vi "TEST_Camera.vi"() -> ()   [LabVIEW 2018]
uses:
  <vilib>/vision/Image Controls.llb/IMAQ Image.ctl
  <vilib>/myRIO/Instrument Drivers/Onboard IO/UART/typedef/VISA Configuration.ctl
  <vilib>/myRIO/Common/Instrument Driver Framework/myRIO v1.0/UART/vis/myRIO v1.0 Close UART.vi
  <vilib>/Instr/_visa.llb/VISA Configure Serial Port (Instr).vi
  <vilib>/Utility/error.llb/Error Cluster From Error Code.vi
  <vilib>/myRIO/Common/Instrument Driver Framework/myRIO v1.0/DIO/vis/myRIO v1.0 Write DIO.vi
  <vilib>/myRIO/Common/Instrument Driver Framework/myRIO v1.0/PWM/vis/myRIO v1.0 Write PWM.vi
  <vilib>/myRIO/Common/Instrument Driver Framework/Utilities/vis/FPGA Ref Manager.vi
  <vilib>/myRIO/Common/Instrument Driver Framework/myRIO v1.0/myRIO v1.0 Reset FPGA.vi
  <vilib>/myRIO/Common/Instrument Driver Framework/myRIO v1.0/IRQ/vis/myRIO v1.0 IRQ Info FGV.vi
  <vilib>/myRIO/Common/Instrument Driver Framework/myRIO v1.0/IRQ/vis/myRIO v1.0 Timer IRQ Info FGV.vi
  <vilib>/myRIO/Common/Instrument Driver Framework/myRIO v1.0/IRQ/vis/myRIO v1.0 ISR Agent.vi
  <vilib>/myRIO/Instrument Drivers/Onboard IO/PWM/PWM.lvlib
  <vilib>/vision/driver/NI_Vision_Acquisition_Software.lvlib
  <vilib>/vision/NI_Vision_Development_Module.lvlib
  <vilib>/myRIO/Instrument Drivers/Utilities/Utilities.lvlib
  <vilib>/myRIO/Instrument Drivers/Onboard IO/DIO/DIO.lvlib
  <vilib>/myRIO/Instrument Drivers/Onboard IO/UART/UART.lvlib
panel:
  in  "RollDetect":bool
  in  "RtF":bool
  in  "State ind":bool
  out "Character Count":u32
  in  "Grounded?":bool
  out "Image 7":T1(plugin-control)
  out "Image Pixels (U8)":u8[][](array[numeric])
  out "Image 6":T1(plugin-control)
  in  "Stop":bool
  out "Image 5":T1(plugin-control)
  out "Y":dbl[](array[numeric])
  out "X":dbl[](array[numeric])
  out "Antal isbjerg":i32
  out "logfile name":path
  in  "logfile base name":string="logfile"
  in  "Color Plane (Color Plane Extraction 1)":i32(ring)=1 items=["Red", "Green", "Blue", "Hue", "Saturation", "Luminance", "Value", "Intensity"]
  in  "Range (Threshold 1)":cluster{"Lower value":sgl, "Upper value":sgl}={"Lower value"=230.0, "Upper value"=255.0}
  in  "Structuring Element (Basic Morphology 1)":i32[][](array[numeric])=[[0, 1, 0], [1, 1, 1], [0, 1, 0]]
  in  "Number of Erosion (Advanced Morphology 1)":i32=12
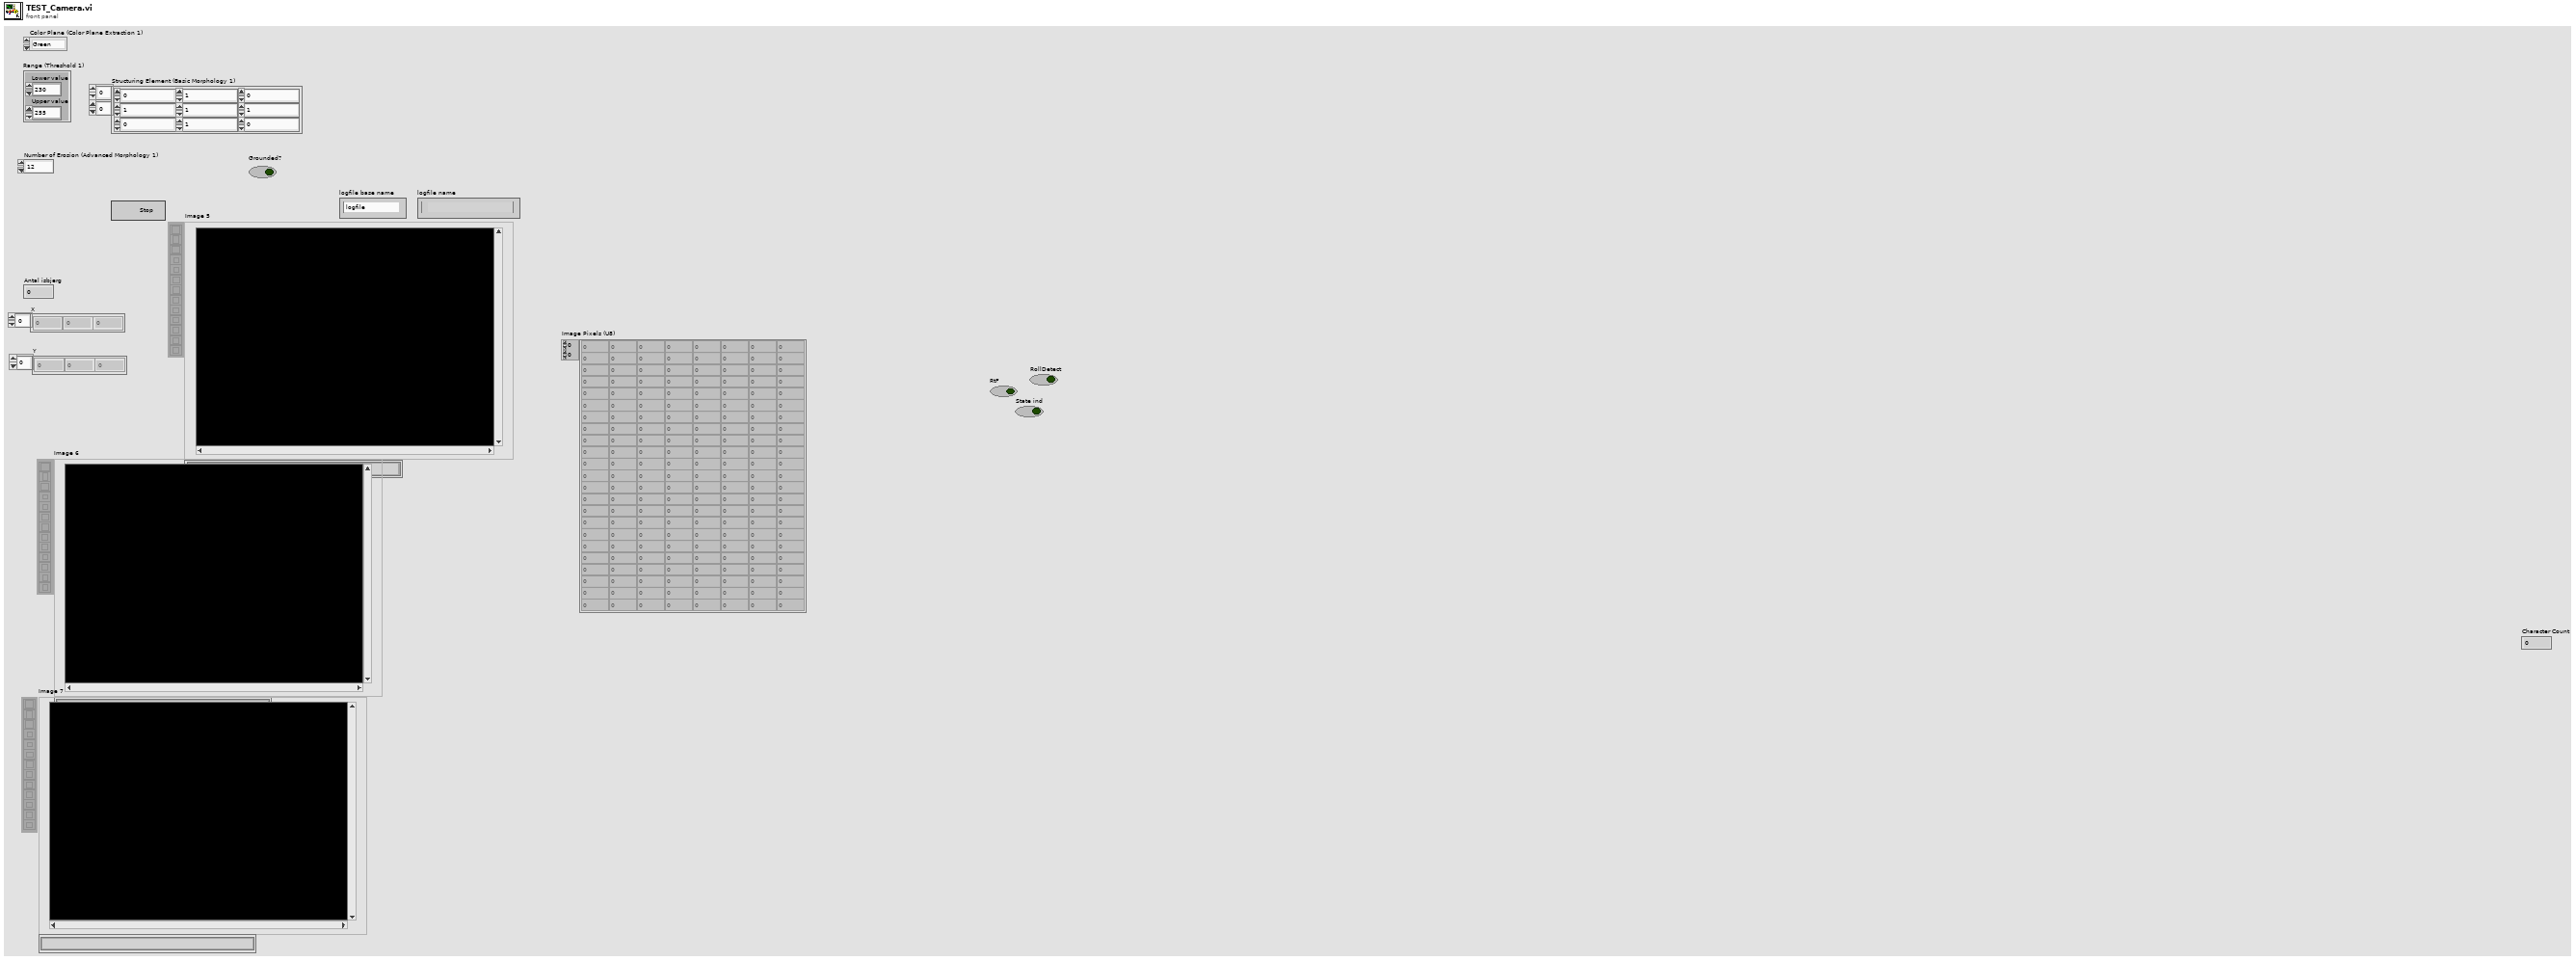
[diagram p1: front panel]
types:
  T1 = typedef "IMAQ Image.ctl" = refnum<image>
  T2 = typedef "DIO.lvlib/DIO Reference.ctl" = cluster{"myRIO Reference":T3, "DIO Channels List":T7}
  T3 = typedef "myRIO Generic Hardware Reference.ctl" = cluster{"myRIO Model":T4, "myRIO Hardware Reference":T5}
  T4 = typedef "Hardware Version Enum.ctl" = enum16{"Unknown", "myRIO-1900", "myRIO-1950", "roboRIO", "NI ELVIS RIO CM", "ELVIS III"}
  T5 = typedef "myRIO v1.0 Reference.ctl" = cluster{"Generic FPGA Reference":T6, "Allow multiple opens":bool}
  T6 = typedef "Generic FPGA Reference.ctl" = refnum<k20>
  T7 = typedef "DIO Channels List.ctl" = T8[]
  T8 = typedef "DIO Channels Enum.ctl" = enum16{"Not Connected", "C/DIO0", "C/DIO1", "C/DIO2", "C/DIO3", "C/DIO4", "C/DIO5", "C/DIO6", "C/DIO7", "A/DIO0", "A/DIO1", "A/DIO2", "A/DIO3", "A/DIO4", "A/DIO5", "A/DIO6", "A/DIO7", "A/DIO8", "A/DIO9", "A/DIO10", "A/DIO11", "A/DIO12", "A/DIO13", "A/DIO14", "A/DIO15", "A/DIO16", "A/DIO17", "A/DIO18", "A/DIO19", "B/DIO0", "B/DIO1", "B/DIO2", "B/DIO3", "B/DIO4", "B/DIO5", "B/DIO6", "B/DIO7", "B/DIO8", "B/DIO9", "B/DIO10", "B/DIO11", "B/DIO12", "B/DIO13", "B/DIO14", "B/DIO15", "B/DIO16", "B/DIO17", "B/DIO18", "B/DIO19", "LED0", "LED1", "LED2", "LED3", "Button0", "DIO/DIO0", "DIO/DIO1", "DIO/DIO2", "DIO/DIO3", "DIO/DIO4", "DIO/DIO5", "DIO/DIO6", "DIO/DIO7", "DIO/DIO8", "DIO/DIO9", "SPI/CS0", "SPI/CS1", "SPI/CS2", "SPI/CS3", "LED RADIO (Green)", "LED RADIO (Red)", "LED COMM (Green)", "LED COMM (Red)", "LED MODE (Green)", "LED MODE (Red)"}
  T9 = typedef "PWM.lvlib/PWM Reference.ctl" = cluster{"myRIO Reference":T3, "PWM Channels Enum":T10, "PWM Configuration":T11}
  T10 = typedef "PWM Channels Enum.ctl" = enum16{"Not Connected", "C/PWM0", "C/PWM1", "A/PWM0", "A/PWM1", "A/PWM2", "A/PWM3", "A/PWM4", "A/PWM5", "A/PWM6", "A/PWM7", "A/PWM8", "A/PWM9", "A/PWM10", "A/PWM11", "A/PWM12", "A/PWM13", "A/PWM14", "A/PWM15", "A/PWM16", "A/PWM17", "A/PWM18", "A/PWM19", "B/PWM0", "B/PWM1", "B/PWM2", "B/PWM3", "B/PWM4", "B/PWM5", "B/PWM6", "B/PWM7", "B/PWM8", "B/PWM9", "B/PWM10", "B/PWM11", "B/PWM12", "B/PWM13", "B/PWM14", "B/PWM15", "B/PWM16", "B/PWM17", "B/PWM18", "B/PWM19", "PWM/PWM0", "PWM/PWM1", "PWM/PWM2", "PWM/PWM3", "PWM/PWM4", "PWM/PWM5", "PWM/PWM6", "PWM/PWM7", "PWM/PWM8", "PWM/PWM9"}
  T11 = typedef "PWM.lvlib/PWM Configuration.ctl" = cluster{"Frequency":dbl, "Duty Cycle":dbl}
  T12 = typedef "Accelerometer.lvlib/Accelerometer Reference.ctl" = cluster{"myRIO Reference":T3, "Accelerometer Channels List":T13, "LSB Weight":dbl}
  T13 = typedef "Accelerometer Channels List.ctl" = T14[]
  T14 = typedef "Accelerometer Channels Enum.ctl" = enum16{"Not Connected", "X-Axis", "Y-Axis", "Z-Axis"}
  T15 = typedef "AI.lvlib/AI Reference.ctl" = cluster{"myRIO Reference":T3, "AI Channels List":T16, "AI Scaling Constants List":T18}
  T16 = typedef "AI Channels List.ctl" = T17[]
  T17 = typedef "AI Channels Enum.ctl" = enum16{"Not Connected", "AudioIn/Left", "AudioIn/Right", "C/AI0", "C/AI1", "A/AI0", "A/AI1", "A/AI2", "A/AI3", "A/AI4", "A/AI5", "A/AI6", "A/AI7", "B/AI0", "B/AI1", "B/AI2", "B/AI3", "B/AI4", "B/AI5", "B/AI6", "B/AI7", "AI/AI0", "AI/AI1", "AI/AI2", "AI/AI3", "A/AI0 (DIFF)", "A/AI1 (DIFF)", "A/AI2 (DIFF)", "A/AI3 (DIFF)", "B/AI0 (DIFF)", "B/AI1 (DIFF)", "B/AI2 (DIFF)", "B/AI3 (DIFF)"}
  T18 = typedef "Analog Scaling Constants List.ctl" = T19[]
  T19 = typedef "Analog Scaling Constants.ctl" = cluster{"LSB Weight (Volts)":dbl, "Offset (Volts)":dbl, "Signed?":bool}
  T20 = typedef "SPI.lvlib/SPI Reference.ctl" = cluster{"myRIO Reference":T3, "SPI Channels Enum":T21, "SPI Configuration":T22}
  T21 = typedef "SPI Channels Enum.ctl" = enum16{"Not Connected", "A/SPI", "B/SPI", "SPI/SPI"}
  T22 = typedef "SPI.lvlib/SPI Configuration.ctl" = cluster{"Frequency [Hz]":dbl, "Clock Phase":T23, "Clock Polarity":T24, "Data Direction":T25, "Frame Length":T26}
  T23 = typedef "SPI Clock Phase.ctl" = enum8{"Leading", "Trailing"}
  T24 = typedef "SPI Clock Polarity.ctl" = enum8{"Low", "High"}
  T25 = typedef "SPI Data Direction.ctl" = enum8{"Most significant bit first", "Least significant bit first"}
  T26 = typedef "SPI Frame Length.ctl" = u8
  T27 = cluster{"B/DIO0 - Stepper Direction":T2, "B/DIO1 - Stepper1 Enable":T2, "B/DIO2 - Stepper2 Enable":T2, "B/DIO3 - Stepper3 Enable":T2, "B/DIO4 - Endstop Stepper1 Top":T2, "B/DIO11 - Endstop Stepper1 Bund":T2, "B/DIO12 - Endstop Stepper2 Top":T2, "B/DIO13 - Endstop Stepper2 Bund":T2, "B/DIO14 - Endstop Stepper3 Top":T2, "B/DIO15 - Endstop Stepper3 Bund":T2, "A/DIO0 - Cooler":T2, "A/DIO1 - Beacon drop (dio1)":T2, "A/DIO2 - Beacon drop (dio0)":T2, "A/DIO3 - QuickRelease (dio1)":T2, "A/DIO4 - QuickRelease (dio0)":T2, "A/DIO11 - LiDAR SPI CS":T2, "B/PWM0 - Stepper":T9, "B/PWM1 - Drill":T9, "A/PWM0 - Servo_Roll":T9, "A/PWM1 - Servo_Yaw":T9, "Acc. X-axis":T12, "Acc. Y-axis":T12, "B/AI0 - Drone Grounded S1 - F3":T15, "A/AI0 - QuickRelease S4 - F4":T15, "B/AI2 - Beacon Drop S5 - F5":T15, "B/AI3 - Begin drilling S3 - F6":T15, "B/AI1 - Gimbal Seach S8 - F8":T15, "A/AI1 - Beacon Wiper":T15, "A/AI2 - QuickRelease Wiper":T15, "A/AI3 - Drill Current":T15, "A/SPI - LiDAR":T20, "B/UART - XBee":refnum<visa-resource-name>, "A/UART - A3 GPS":refnum<visa-resource-name>, "RIO Flashing LEDs":T2}
  T28 = enum32{"AutoM", "Close", "Dilate", "Erode", "Gradient", "Gradient out", "Gradient in", "Hit miss", "Open", "PClose", "POpen", "Thick", "Thin"}
  T29 = typedef "UART.lvlib/VISA Configuration.ctl" = cluster{"baud rate (9600)":u32, "data bits (8)":u16, "parity (0:none)":enum16{"None", "Odd", "Even", "Mark", "Space"}, "stop bits (10: 1 bit)":u16, "flow control (0:none)":u16, "termination char\n(0xA = '\\n' = LF) ":u8, "Enable Termination\nChar (T)":bool, "timeout (10sec)":u32}
  T30 = typedef "Image Type" = u32
  T31 = typedef "IMAQdx.ctl" = refnum<k21>
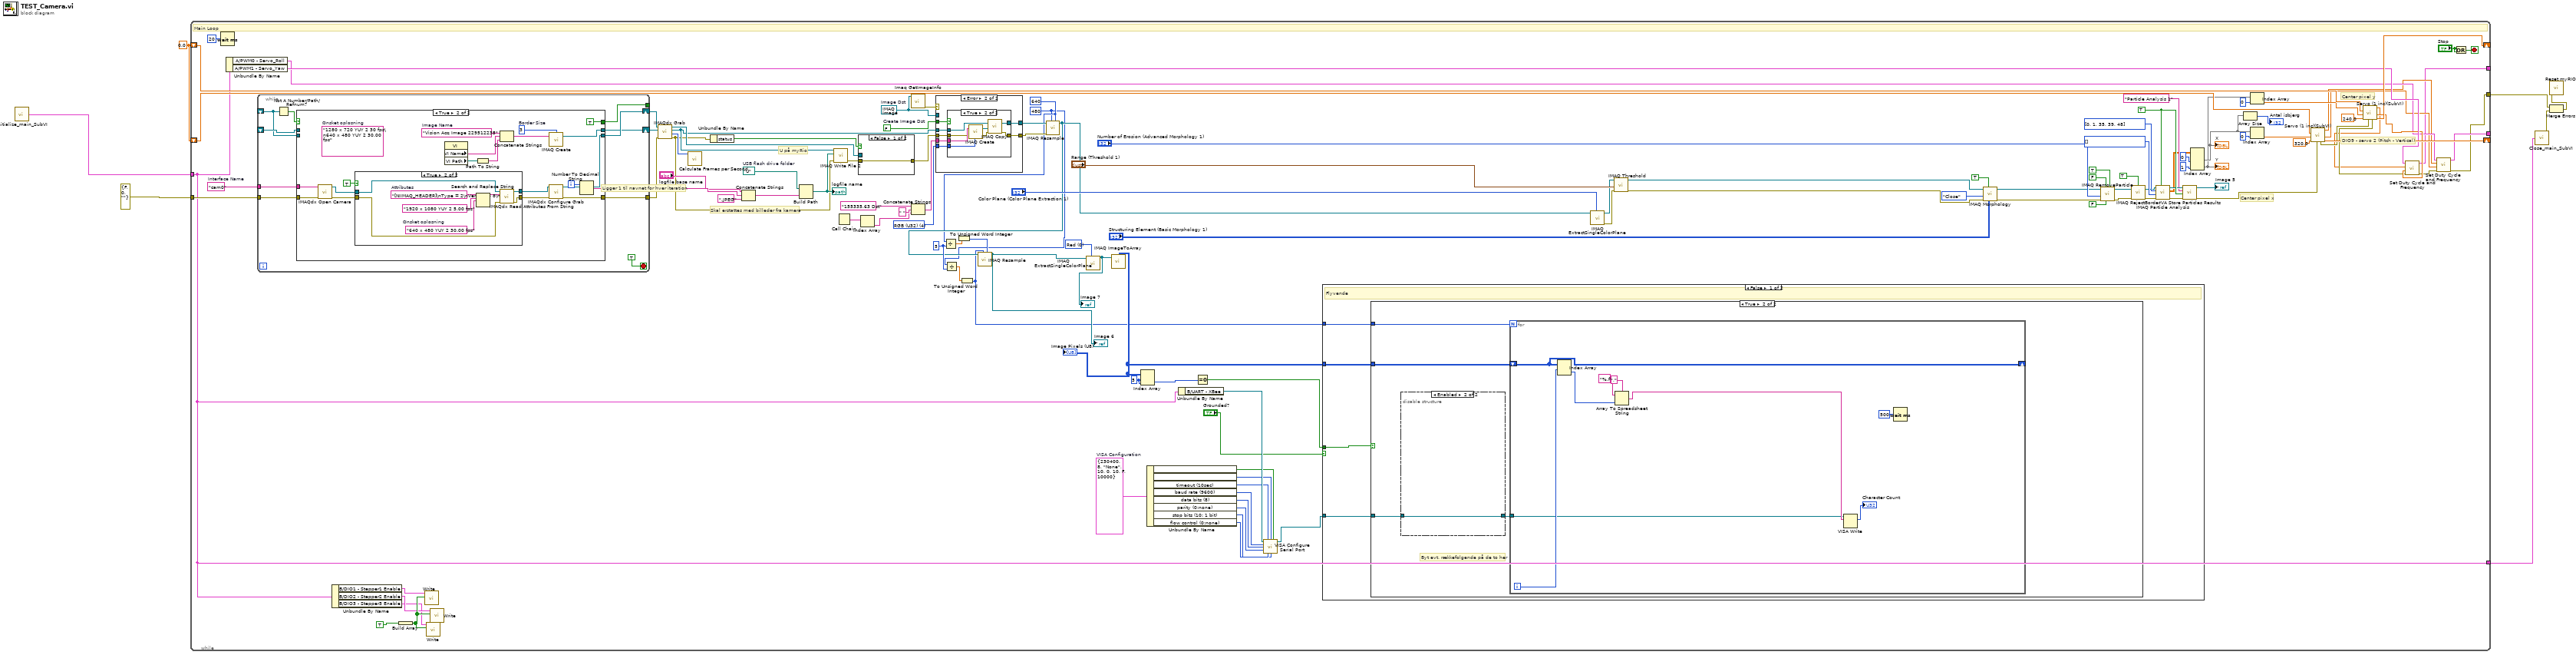
[diagram p0: block diagram]
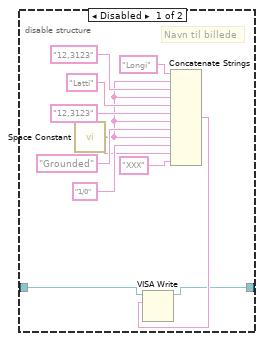
[diagram p3: hidden frame]
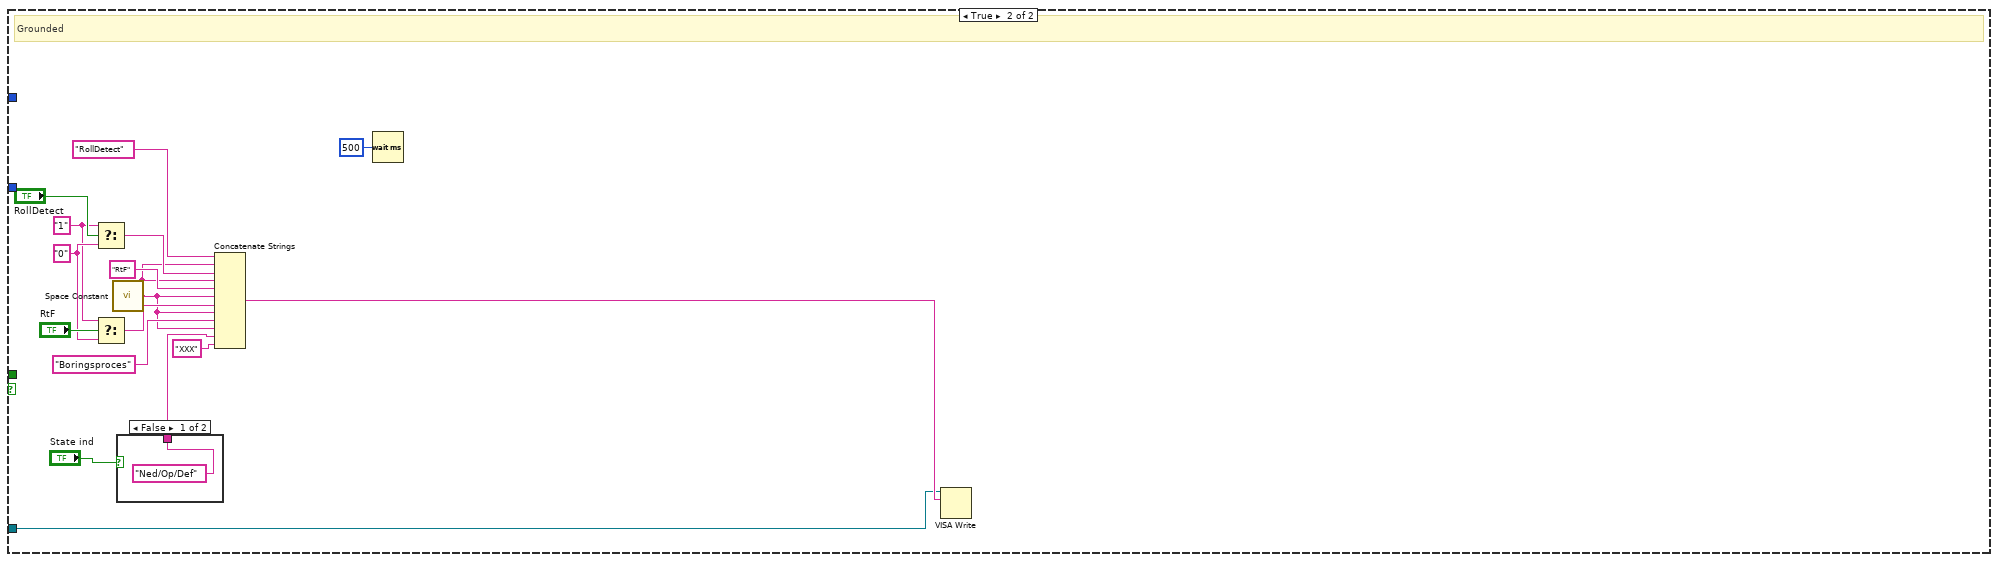
[diagram p4: hidden frame]
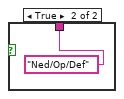
[diagram p5: hidden frame]
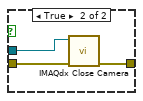
[diagram p6: hidden frame]
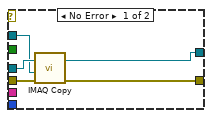
[diagram p9: hidden frame]
diagram:
  w6 = 0.0 ("Position 2")
  n1 = call "Initialize_main_SubVI.vi"() -> ("output cluster"=w1:T27)
  n2 = while {
    shift-right: [w95] -> _
    shift-left: w6 -> [w98]
    shift-right: [w110] -> _
    shift-left: w6 -> [w111]
    tunnel: errorcluster {"status"=FALSE, "code"=0, "source"=""} ("error out") -> [w112]
    tunnel: w1 -> [w23]
    tunnel: [w37] -> w3
    tunnel: [w46] -> _
    tunnel: [w45] -> _
    tunnel: [w23] -> w5
    i -> [w85]
    stop <- w129 stop-if-true
    w13 = T29 {"baud rate (9600)"=230400, "data bits (8)"=8, "parity (0:none)"=enum."None", "stop bits (10: 1 bit)"=10, "flow control (0:none)"=0, "termination char\n(0xA = '\\n' = LF) "=10, "Enable Termination\nChar (T)"=FALSE, "timeout (10sec)"=10000}  # VISA Configuration
    w25 = 5 ("index (row)")
    w34 = 0 items=["Red", "Green", "Blue", "Hue", "Saturation", "Luminance", "Value", "Intensity"] ("Color Plane")
    w35 = u16 5 ("y")
    w29 = u32 640 ("Width")
    w28 = u32 480 ("Height")
    w63 = i32[] [] items=["Center of Mass X", "Center of Mass Y", "First Pixel X", "First Pixel Y", "Bounding Rect Left", "Bounding Rect Top", "Bounding Rect Right", "Bounding Rect Bottom", "Max Feret Diameter Start X", "Max Feret Diameter Start Y", "Max Feret Diameter End X", "Max Feret Diameter End Y", "Max Horiz. Segment Length Left", "Max Horiz. Segment Length Right", "Max Horiz. Segment Length Row", "-", "Bounding Rect Width", "Bounding Rect Height", "Bounding Rect Diagonal", "Perimeter", "Convex Hull Perimeter", "Holes' Perimeter", "Max Feret Diameter", "Equivalent Ellipse Major Axis", "Equivalent Ellipse Minor Axis", "Equivalent Ellipse Minor Axis (Feret)", "Equivalent Rect Long Side", "Equivalent Rect Short Side", "Equivalent Rect Diagonal", "Equivalent Rect Short Side (Feret)", "Average Horiz. Segment Length", "Average Vert. Segment Length", "Hydraulic Radius", "Waddel Disk Diameter", "-", "Area", "Holes' Area", "Particle & Holes' Area", "Convex Hull Area", "Image Area", "-", "Number of Holes", "Number of Horiz. Segments", "Number of Vert. Segments", "-", "Orientation", "Max Feret Diameter Orientation", "-", "% Area/Image Area", "% Area/(Particle & Holes' Area)", "Ratio of Equivalent Ellipse Axes", "Ratio of Equivalent Rect Sides", "-", "Elongation Factor", "Compactness Factor", "Heywood Circularity Factor", "Type Factor", "-", "Sum X", "Sum Y", "Sum XX", "Sum XY", "Sum YY", "Sum XXX", "Sum XXY", "Sum XYY", "Sum YYY", "-", "Moment of Inertia XX", "Moment of Inertia XY", "Moment of Inertia YY", "Moment of Inertia XXX", "Moment of Inertia XXY", "Moment of Inertia XYY", "Moment of Inertia YYY", "Norm. Moment of Inertia XX", "Norm. Moment of Inertia XY", "Norm. Moment of Inertia YY", "Norm. Moment of Inertia XXX", "Norm. Moment of Inertia XXY", "Norm. Moment of Inertia XYY", "Norm. Moment of Inertia YYY", "Hu Moment 1", "Hu Moment 2", "Hu Moment 3", "Hu Moment 4", "Hu Moment 5", "Hu Moment 6", "Hu Moment 7"] ("Real-World Measurements")
    w64 = i32[] [0, 1, 35, 39, 48] items=["Center of Mass X", "Center of Mass Y", "First Pixel X", "First Pixel Y", "Bounding Rect Left", "Bounding Rect Top", "Bounding Rect Right", "Bounding Rect Bottom", "Max Feret Diameter Start X", "Max Feret Diameter Start Y", "Max Feret Diameter End X", "Max Feret Diameter End Y", "Max Horiz. Segment Length Left", "Max Horiz. Segment Length Right", "Max Horiz. Segment Length Row", "-", "Bounding Rect Width", "Bounding Rect Height", "Bounding Rect Diagonal", "Perimeter", "Convex Hull Perimeter", "Holes' Perimeter", "Max Feret Diameter", "Equivalent Ellipse Major Axis", "Equivalent Ellipse Minor Axis", "Equivalent Ellipse Minor Axis (Feret)", "Equivalent Rect Long Side", "Equivalent Rect Short Side", "Equivalent Rect Diagonal", "Equivalent Rect Short Side (Feret)", "Average Horiz. Segment Length", "Average Vert. Segment Length", "Hydraulic Radius", "Waddel Disk Diameter", "-", "Area", "Holes' Area", "Particle & Holes' Area", "Convex Hull Area", "Image Area", "-", "Number of Holes", "Number of Horiz. Segments", "Number of Vert. Segments", "-", "Orientation", "Max Feret Diameter Orientation", "-", "% Area/Image Area", "% Area/(Particle & Holes' Area)", "Ratio of Equivalent Ellipse Axes", "Ratio of Equivalent Rect Sides", "-", "Elongation Factor", "Compactness Factor", "Heywood Circularity Factor", "Type Factor", "-", "Sum X", "Sum Y", "Sum XX", "Sum XY", "Sum YY", "Sum XXX", "Sum XXY", "Sum XYY", "Sum YYY", "-", "Moment of Inertia XX", "Moment of Inertia XY", "Moment of Inertia YY", "Moment of Inertia XXX", "Moment of Inertia XXY", "Moment of Inertia XYY", "Moment of Inertia YYY", "Norm. Moment of Inertia XX", "Norm. Moment of Inertia XY", "Norm. Moment of Inertia YY", "Norm. Moment of Inertia XXX", "Norm. Moment of Inertia XXY", "Norm. Moment of Inertia XYY", "Norm. Moment of Inertia YYY", "Hu Moment 1", "Hu Moment 2", "Hu Moment 3", "Hu Moment 4", "Hu Moment 5", "Hu Moment 6", "Hu Moment 7"] ("Pixel Measurements")
    w61 = TRUE ("Connectivity 4/8 (8)")
    w84 = path "U:/"  # USB flash drive folder
    w118 = "cam0"  # Interface Name
    w128 = T1 refnum  # Image Dst
    w120 = T30 4 items=["Grayscale (U8)", "Grayscale (I16)", "Grayscale (SGL)", "Complex (CSG)", "RGB (U32)", "HSL (U32)", "RGB (U64)", "Grayscale (U16)"] ("Image Dst Type")
    w126 = FALSE  # Create Image Dst
    # "U på myRio"
    # "Ligger 1 til navnet for hver iteration"
    # "Skal erstattes med billeder fra kamera"
    # "Center pixel y"
    # "Center pixel x"
    # "DIO9 - servo 2 (Pitch - Vertical)"
    # "Main Loop"
    n3 = Wait (ms)(milliseconds to wait=u32 20) -> ()  [unwired: 1 out]
    n4 = Unbundle By Name(w23) -> ("A/PWM0 - Servo_Roll"=w49:T9, "A/PWM1 - Servo_Yaw"=w51:T9)
    n5 = while "While Loop_template0" {
      shift-right: [w190] -> w113
      shift-left: _ -> [w183]
      tunnel: [w189] -> w119
      tunnel: w112 -> [w188]
      shift-right: [w186] -> w114
      shift-left: _ -> [w185]
      tunnel: w118 -> [w184]
      tunnel: [w181] -> _
      stop <- TRUE ("_template0") stop-if-true
      n6 = Not A Number/Path/Refnum?(number/path/refnum=w183) -> (NaN/Path/Refnum?=w182:bool)
      n7 = case "Case Structure_template0" shown="True" w182 {
        tunnel: [w193 w209] -> w190
        tunnel: w183 -> [w193 _]
        tunnel: [w192 w208] -> w189
        tunnel: w188 -> [w192 w210]
        tunnel: [w191 w207] -> w186
        tunnel: w185 -> [w191 _]
        tunnel: w184 -> [_ w198]
        tunnel: [_ TRUE] -> w181
        frame False {
        }
        frame True {
          (unwired) "1280 x 720 YUY 2 30 fps\n640 x 480 YUY 2 30.00 fps"  # Ønsket opløsning
          w195 = 3  # Border Size
          w202 = "Vision Acq Image 229512235"  # Image Name
          n8 = call <vilib>:"IMAQdx Open Camera.vi"("error in"=w210, "Session In"=w198) -> ("error out"=w200:errorcluster, "Session Out"=w201:T31)  [unwired: 1 in, 7 out]
          n9 = case shown="True" TRUE ("Init Attributes") {
            tunnel: w201 -> [w212 w220]
            tunnel: w200 -> [w211 w219]
            tunnel: [w212 w218] -> w194
            tunnel: [w211 w217] -> w199
            frame False {
            }
            frame True {
              w213 = "640 x 480 YUY 2 30.00 fps"  # Ønsket opløsning
              w216 = "[NIIMAQ_HEADER]\nType = 2\nVersion = 8\n\n[CAMERA_DATA]\nAcquisitionAttributes::Bayer::Algorithm = \"Bilinear\"\nAcquisitionAttributes::Bayer::GainB = \"1\"\nAcquisitionAttributes::Bayer::GainG = \"1\"\nAcquisitionAttributes::Bayer::GainR = \"1\"\nAcquisitionAttributes::Bayer::Pattern = \"Use hardware value\"\nAcquisitionAttributes::BitsPerPixel = \"Use hardware value\"\nAcquisitionAttributes::HardwareMaximumQueuedBufferCount = \"1000\"\nAcquisitionAttributes::HardwareRequeueBufferListThreshold = \"50\"\nAcquisitionAttributes::IgnoreFirstFrame = \"false\"\nAcquisitionAttributes::ImageDecoderCopyMode = \"Auto\"\nAcquisitionAttributes::OutputImageType = \"Auto\"\nAcquisitionAttributes::OverwriteMode = \"Get Newest\"\nAcquisitionAttributes::PixelSignedness = \"Use hardware value\"\nAcquisitionAttributes::ReceiveTimestampMode = \"None\"\nAcquisitionAttributes::ShiftPixelBits = \"false\"\nAcquisitionAttributes::SwapPixelBytes = \"false\"\nAcquisitionAttributes::Timeout = \"5000\"\nAcquisitionAttributes::VideoMode = \"1920 x 1080 YUY 2 5.00 fps\"\nCameraAttributes::BacklightCompensation::Mode = \"Manual\"\nCameraAttributes::BacklightCompensation::Value = \"0\"\nCameraAttributes::Brightness::Mode = \"Manual\"\nCameraAttributes::Brightness::Value = \"168\"\nCameraAttributes::Contrast::Mode = \"Manual\"\nCameraAttributes::Contrast::Value = \"5\"\nCameraAttributes::Exposure::Mode = \"AutoAperaturePriority\"\nCameraAttributes::Focus::Mode = \"Auto\"\nCameraAttributes::Pan::Mode = \"Manual\"\nCameraAttributes::Pan::Value = \"0\"\nCameraAttributes::PowerLineFrequency::Mode = \"60Hz\"\nCameraAttributes::Saturation::Mode = \"Manual\"\nCameraAttributes::Saturation::Value = \"103\"\nCameraAttributes::Sharpness::Mode = \"Manual\"\nCameraAttributes::Sharpness::Value = \"25\"\nCameraAttributes::Tilt::Mode = \"Manual\"\nCameraAttributes::Tilt::Value = \"0\"\nCameraAttributes::WhiteBalance::Mode = \"Auto\"\nCameraAttributes::Zoom::Mode = \"Manual\"\nCameraAttributes::Zoom::Value = \"0\"\n"  # Attributes
              n10 = Search and Replace String(input string=w216, search string="1920 x 1080 YUY 2 5.00 fps", replace string=w213) -> (result string=w214:string)  [unwired: 5 in, 3 out]
              n11 = call <vilib>:"IMAQdx Read Attributes From String.vi"("error in"=w219, "Attributes String In"=w214, "Session In"=w220) -> ("error out"=w217:errorcluster, "Session Out"=w218:T31)  [unwired: 7 out]
            }
          }
          n12 = property class="VI"() -> ("VI Name"=w205:string, "VI Path"=w206:path)  [unwired: 2 in, 2 out]
          n13 = Path To String(path=w206) -> (string=w204:string)
          n14 = Concatenate Strings(w202, w205, w204) -> (w203:string)
          n15 = call "IMAQ Create"("Border Size"=w195, "Image Name"=w203) -> ("New Image"=w207:T1)  [unwired: 2 in, 2 out]
          n16 = call <vilib>:"IMAQdx Configure Grab.vi"("error in"=w199, "Session In"=w194) -> ("error out"=w208:errorcluster, "Session Out"=w209:T31)  [unwired: 8 out]
        }
      }
    }
    n17 = Unbundle By Name(w23) -> ("B/DIO1 - Stepper1 Enable"=w42:T2, "B/DIO2 - Stepper2 Enable"=w41:T2, "B/DIO3 - Stepper3 Enable"=w40:T2)
    n18 = Build Array(TRUE) -> (w43:bool[])
    n19 = call <vilib>:"Write.vi"("Values"=w43, "DIO Ref In"=w42) -> ()  [unwired: 7 in, 2 out]
    n20 = call <vilib>:"Write.vi"("Values"=w43, "DIO Ref In"=w40) -> ()  [unwired: 7 in, 2 out]
    n21 = call <vilib>:"Write.vi"("Values"=w43, "DIO Ref In"=w41) -> ()  [unwired: 7 in, 2 out]
    n22 = Number To Decimal String(number=w85) -> (decimal integer string=w90:string)  [unwired: 1 in]
    n23 = call <vilib>:"IMAQdx Grab.vi"("error in"=w119, "Image In"=w114, "Session In"=w113) -> ("error out"=w87:errorcluster, "Buffer Number Out"=w117:u32, "Image Out"=w88:T1, "Session Out"=w116:T31)  [unwired: 1 in, 4 out]
    n24 = call <vilib>:"Calculate Frames per Second.vi"("Buffer Number"=w117) -> ()  [unwired: 2 in, 9 out]
    n25 = Unbundle By Name(w87) -> ("status"=w107:bool)
    n26 = Concatenate Strings "Concatenate Strings"("logfile base name", w90, ".JPEG" ("string")) -> (w92:string)
    n27 = Build Path(base path=w84, name or relative path=w92) -> (appended path=w93:path)
    "logfile name" <- w93
    n28 = call-poly "IMAQ Write File 2"("error in (no error)"=w87, "File Path"=w93, "Image"=w88) -> ("error out"=w86:errorcluster)  [unwired: 7 in, 1 out]
    n29 = Call Chain() -> (call chain=w125:string[])
    n30 = case "Case Structure_template1" shown="False" w107 {
      tunnel: [w177 w179] -> w115
      tunnel: w86 -> [w177 w180]
      tunnel: w116 -> [_ w178]
      frame False {
      }
      frame True {
        n31 = call <vilib>:"IMAQdx Close Camera.vi"("error in"=w180, "Session In"=w178) -> ("error out"=w179:errorcluster)  [unwired: 9 out]
      }
    }
    n32 = Index Array(array=w125) -> (element=w123:string)  [unwired: 1 in]
    n33 = call "Imaq GetImageInfo"("Image"=w128) -> ("error out"=w127:errorcluster)  [unwired: 1 in, 9 out]
    n34 = Concatenate Strings("155335,63 Dst" ("Image Dst Name"), " ", w123) -> (w121:string)
    n35 = case shown="Error" w127 {
      tunnel: [w225 w229] -> w54
      tunnel: [w224 w228] -> w53
      tunnel: w88 -> [w223 w230]
      tunnel: w115 -> [w222 w226]
      tunnel: w128 -> [w221 _]
      tunnel: w121 -> [_ w232]
      tunnel: w120 -> [_ w231]
      tunnel: w126 -> [_ w227]
      frame No Error {
        n36 = call "IMAQ Copy"("error in (no error)"=w222, "Image Dst"=w221, "Image Src"=w223) -> ("error out"=w224:errorcluster, "Image Dst Out"=w225:T1)  [unwired: 3 out]
      }
      frame Error {
        n37 = case shown="True" w227 {
          tunnel: w232 -> [_ w242]
          tunnel: w231 -> [_ w241]
          tunnel: w230 -> [w234 w239]
          tunnel: [w234 w238] -> w229
          tunnel: [w233 w237] -> w228
          tunnel: w226 -> [w233 w235]
          frame False {
          }
          frame True {
            n38 = call "IMAQ Create"("Image Name"=w242, "Image Type"=w241, "error in (no error)"=w235) -> ("New Image"=w240:T1, "error out"=w236:errorcluster)  [unwired: 1 in, 1 out]
            n39 = call "IMAQ Copy"("error in (no error)"=w236, "Image Dst"=w240, "Image Src"=w239) -> ("error out"=w237:errorcluster, "Image Dst Out"=w238:T1)  [unwired: 3 out]
          }
        }
      }
    }
    n40 = Divide(x=w29, y=w35) -> (x/y=w32:dbl)
    n41 = Divide(x=w28, y=w35) -> (x/y=w33:dbl)
    n42 = To Unsigned Word Integer(number=w32) -> (unsigned 16bit integer=w31:u16)
    n43 = To Unsigned Word Integer(number=w33) -> (unsigned 16bit integer=w10:u16)
    n44 = call "IMAQ Resample"("X Resolution"=w29, "Y Resolution"=w28, "error in (no error)"=w53, "Image Src"=w54) -> ("Image Dst Out"=w30:T1)  [unwired: 6 in, 1 out]
    n45 = call "IMAQ Resample"("X Resolution"=w31, "Y Resolution"=w10, "Image Src"=w30) -> ("Image Dst Out"=w27:T1)  [unwired: 7 in, 1 out]
    "Image 6" <- w27
    n46 = call "IMAQ ExtractSingleColorPlane"("Color Plane"=w34, "Image Src"=w27) -> ("Image Dst Out"=w26:T1)  [unwired: 8 in, 1 out]
    "Image 7" <- w26
    n47 = call "IMAQ ImageToArray"("Image"=w26) -> ("Image Pixels (U8)"=w11:u8[][])  [unwired: 3 in, 4 out]
    "Image Pixels (U8)" <- w11
    n48 = Index Array(array=w11, index (row)=w25, index (col)=w25) -> (element=w24:u8)
    n49 = Unbundle By Name(w13) -> ("Enable Termination\nChar (T)"=w14:bool, "termination char\n(0xA = '\\n' = LF)"=w15:u8, "timeout (10sec)"=w16:u32, "baud rate (9600)"=w21:u32, "data bits (8)"=w20:u16, "parity (0:none)"=w19:enum16{"None", "Odd", "Even", "Mark", "Space"}, "stop bits (10: 1 bit)"=w18:u16, "flow control (0:none)"=w17:u16)
    n50 = Unbundle By Name(w23) -> ("B/UART - XBee"=w22:refnum<visa-resource-name>)
    n51 = Equal To 0?(x=w24) -> (x = 0?=w8:bool)
    n52 = call-poly "VISA Configure Serial Port"("VISA resource name"=w22, "timeout (10sec)"=w16, "termination char\n(0xA = '\\n' = LF)"=w15, "Enable Termination\nChar (T)"=w14, "baud rate (9600)"=w21, "data bits (8)"=w20, "parity (0:none)"=w19, "stop bits (10: 1 bit)"=w18, "flow control (0:none)"=w17) -> ("VISA resource name out"=w12:refnum<visa-resource-name>)  [unwired: 5 in, 1 out]
    n53 = case shown="False" "Grounded?" {
      tunnel: w11 -> [w133 _]
      tunnel: w10 -> [w132 _]
      tunnel: w8 -> [w131 _]
      tunnel: w12 -> [w130 w162]
      frame False {
        # "Flyvende"
        n54 = case shown="True" w131 {
          tunnel: w133 -> [_ w137]
          tunnel: w132 -> [_ w136]
          tunnel: w130 -> [_ w134]
          frame False {
          }
          frame True {
            # "Byt evt. rækkefølgende på de to her"
            n55 = disable-structure shown="Enabled" {
              disable-tunnel: [w139 w149] -> w135
              disable-tunnel: w134 -> [w138 w149]
              frame Disabled {
                # "Navn til billede"
                n56 = call <vilib>:"Space Constant.vi"() -> ("String"=w141:string)
                n57 = Concatenate Strings("Longi", w141, "12,3123" ("string"), w141, "Latti", "12,3123" ("string"), w141, "Grounded", w141, "1/0", w141, "XXX" ("string")) -> (w144:string)
                n58 = VISA Write(VISA resource name=w138, write buffer=w144) -> (VISA resource name out=w139:refnum<visa-resource-name>)  [unwired: 1 in, 2 out]
              }
              frame Enabled {
              }
            }
            n59 = for {
              N: w136 -> [_]
              shift-right: [w157] -> _
              shift-left: w137 -> [w157]
              tunnel: w135 -> [w150]
              i -> [w158]
              n60 = Index Array(array=w157, index (row)=w158) -> (element=w155:u8[])  [unwired: 1 in]
              n61 = Array To Spreadsheet String(delimiter (Tab)=",", array=w155, 3:"%.f" ("format string")) -> (spreadsheet string=w152:string)
              n62 = VISA Write(VISA resource name=w150, write buffer=w152) -> (return count=→"Character Count":u32)  [unwired: 1 in, 2 out]
              n63 = Wait (ms)(milliseconds to wait=u32 500) -> ()  [unwired: 1 out]
            }
          }
        }
      }
      frame True {
        w168 = "0" ("string")
        w167 = "1" ("string")
        # "Grounded"
        n64 = Select(t=w167, s="RollDetect", f=w168) -> (s? t:f=w172:string)
        n65 = Select(t=w167, s="RtF", f=w168) -> (s? t:f=w166:string)
        n66 = call <vilib>:"Space Constant.vi"() -> ("String"=w164:string)
        n67 = case shown="False" "State ind" {
          tunnel: ["Ned/Op/Def" ("string") "Ned/Op/Def" ("string")] -> w160
          frame False {
          }
          frame True {
          }
        }
        n68 = Concatenate Strings("RollDetect" ("string"), w164, w172, w164, "RtF" ("string"), w164, w166, w164, "Boringsproces" ("string"), w164, w160, "XXX" ("string")) -> (w174:string)
        n69 = Wait (ms)(milliseconds to wait=u32 500) -> ()  [unwired: 1 out]
        n70 = VISA Write(VISA resource name=w162, write buffer=w174) -> ()  [unwired: 1 in, 3 out]
      }
    }
    n71 = call "IMAQ ExtractSingleColorPlane"("Color Plane"="Color Plane (Color Plane Extraction 1)", "Image Src"=w30) -> ("error out"=w82:errorcluster, "Image Dst Out"=w80:T1)  [unwired: 2 in, 6 out]
    n72 = call "IMAQ Threshold"("error in (no error)"=w82, "Range"="Range (Threshold 1)", "Image Src"=w80) -> ("error out"=w79:errorcluster, "Image Dst Out"=w75:T1)  [unwired: 3 in, 4 out]
    n73 = call "IMAQ Morphology"("Structuring Element"="Structuring Element (Basic Morphology 1)", "Square/Hexa (Square)"=TRUE, "error in (no error)"=w79, "Operation"=T28."Close", "Image Src"=w75) -> ("error out"=w74:errorcluster, "Image Dst Out"=w69:T1)  [unwired: 2 in, 3 out]
    n74 = call "IMAQ RemoveParticle"("Connectivity 4/8 (8)"=TRUE, "Low Pass/High Pass (Low)"=FALSE, "Square/Hexa (Square)"=FALSE, "error in (no error)"=w74, "Number of Erosion"="Number of Erosion (Advanced Morphology 1)", "Image Src"=w69) -> ("error out"=w68:errorcluster, "Image Dst Out"=w66:T1)  [unwired: 1 in, 3 out]
    n75 = call "IMAQ RejectBorder"("error in (no error)"=w68, "Image Src"=w66, "Connectivity 4/8 (8)"=TRUE) -> ("error out"=w65:errorcluster, "Image Dst Out"=w62:T1)  [unwired: 1 in, 2 out]
    n76 = call "IMAQ Particle Analysis"("Connectivity 4/8 (8)"=w61, "error in (no error)"=w65, "Real-World Measurements"=w63, "Pixel Measurements"=w64, "Image"=w62) -> ("error out"=w58:errorcluster, "Particle Measurements (Pixels)"=w55:dbl[][], "Image Out (duplicate)"=w60:T1)  [unwired: 4 out]
    n77 = call <vilib>:"IVA Store Particles Results.vi"("error in (no error)"=w58, "Connectivity 4/8 (8)"=w61, "Step Name"="Particle Analysis 1", "Image in"=w60) -> ("error out"=w56:errorcluster, "Image dup"=→"Image 5":T1)  [unwired: 6 out]
    n78 = Index Array(array=w55, index (col) #1=0 ("index (col)"), index (col) #2=1 ("index (col)")) -> (element #1=w102:dbl[], element #2=w99:dbl[])  [unwired: 2 in]
    "Y" <- w99
    "X" <- w102
    n79 = Array Size(array=w102) -> (size(s)=→"Antal isbjerg":i32)
    n80 = Index Array(array=w99, index=0) -> (element=w94:dbl)
    n81 = Index Array(array=w102, index=0) -> (element=w101:dbl)
    n82 = call "Servo (1 inc)(SubVI).vi"("error constant 2"=w56, "Center pixel"=320.0 ("Center pixel 2"), "Pixel value"=w101, "Position."=w111) -> ("Position 2"=w110:dbl, "freq [Hz]"=w47:dbl, "Duty"=w48:dbl, "error constant"=w96:errorcluster)  [unwired: 3 in, 1 out]
    n83 = call "Servo (1 inc)(SubVI).vi"("error constant 2"=w96, "Center pixel"=240.0, "Pixel value"=w94, "Position."=w98) -> ("Position 2"=w95:dbl, "freq [Hz]"=w50:dbl, "Duty"=w36:dbl, "error constant"=w39:errorcluster)  [unwired: 3 in, 1 out]
    n84 = call <vilib>:"Set Duty Cycle and Frequency.vi"("error in (no error)"=w39, "Frequency [Hz]"=w50, "Duty Cycle"=w36, "PWM Ref In"=w51) -> ("error out"=w38:errorcluster, "PWM Ref Out"=w46:T9)  [unwired: 5 in]
    n85 = call <vilib>:"Set Duty Cycle and Frequency.vi"("error in (no error)"=w38, "Frequency [Hz]"=w47, "Duty Cycle"=w48, "PWM Ref In"=w49) -> ("error out"=w37:errorcluster, "PWM Ref Out"=w45:T9)  [unwired: 5 in]
    n86 = Or(x="Stop", y="Stop") -> (x .or. y?=w129:bool)
  }
  n87 = call "Close_main_SubVI.vi"("output cluster"=w5) -> ("error constant"=w4:errorcluster)
  n88 = Merge Errors(w3, w4) -> (w2:errorcluster)
  n89 = call <vilib>:"Reset myRIO.vi"("error in (no error)"=w2) -> ()  [unwired: 10 in, 1 out]
